vi "DBO.vi"(1 "H":dbl[][](array[numeric]), 2 "x":dbl) -> (0 "y":dbl)   [LabVIEW 2011]
uses:
  <vilib>/imath/engines/lvmath2/RunTimeEngine/ErrorHandling/NIMS_Finalize Error.vi
  <vilib>/imath/engines/lvmath2/RunTimeEngine/BuiltInFunctions/size/NIMS_I32=size(GM,I32).vi
  <instcachedir>/0/NIMS_I32=size(GM,I32)_C888250C35F946008B07D98778967D76.lvgen/NIMS_I32=size(GM,I32)_C888250C35F946008B07D98778967D76_004.vi
  <vilib>/imathl/engines/lvmath/Functions/Error Handling/Create Error.vi
  <vilib>/imath/engines/lvmath2/RunTimeEngine/CommandStatement/NIMS_CommandStatement_MaskErr.vi
  <vilib>/imath/engines/lvmath2/RunTimeEngine/VariableToken/NIMS_VariableToken_CondDefined.vi
  <instcachedir>/0/NIMS_VariableToken_CondDefined_D30D2F4D3CE04567BC79CC35D27951F7.lvgen/NIMS_VariableToken_CondDefined_D30D2F4D3CE04567BC79CC35D27951F7_003.vi
  <vilib>/imath/engines/lvmath/Functions/Error Handling/MergeErrorsWrapper.vi
  <vilib>/imath/engines/lvmath2/RunTimeEngine/NodeEndStatement/NIMS_NodeEndStatement_Output.vi
  <instcachedir>/0/NIMS_NodeEndStatement_Output_53EC0D466D134D7ABD903AC30B43404B.lvgen/NIMS_NodeEndStatement_Output_53EC0D466D134D7ABD903AC30B43404B_001.vi
  <vilib>/imath/engines/lvmath2/RunTimeEngine/VariableToken/Read/NIMS_Get Elements - SorM(_,_) - Check - Check.vi
  <instcachedir>/0/NIMS_Get Elements - SorM(_,_) - Check - Check_DA1E252EAB634D989357E7C72E8137F5.lvgen/NIMS_Get Elements - SorM(_,_) - Check - Check_DA1E252EAB634D989357E7C72E8137F5_001.vi
  C:/Documents and Settings/yna/My Documents/LabVIEW Data/MathScriptVIs/MCStatic_285220864_6d3d3726c5e701717503ad0a97b9c04b.vi
  <instcachedir>/0/MCStatic_285220864_6d3d3726c5e701717503ad0a97b9c04b_95A5838EAFCD4223B404CBD5C4A8267C.lvgen/MCStatic_285220864_6d3d3726c5e701717503ad0a97b9c04b_95A5838EAFCD4223B404CBD5C4A8267C_000.vi
  C:/Documents and Settings/yna/My Documents/LabVIEW Data/MathScriptVIs/MCStatic_285220864_904684f4bc757d8a144c5b0c95be3f99.vi
  <instcachedir>/0/MCStatic_285220864_904684f4bc757d8a144c5b0c95be3f99_DB46245F63EA4693B729F1F383828BBE.lvgen/MCStatic_285220864_904684f4bc757d8a144c5b0c95be3f99_DB46245F63EA4693B729F1F383828BBE_000.vi
  <vilib>/imath/engines/lvmath2/RunTimeEngine/BuiltInFunctions/min/2 inputs/NIMS_min(RG,RG)-no size check.vi
  <instcachedir>/0/NIMS_min(RG,RG)-no size check_7F67BAB91AFC452D9517D2EA1C8F5F88.lvgen/NIMS_min(RG,RG)-no size check_7F67BAB91AFC452D9517D2EA1C8F5F88_001.vi
  <vilib>/imath/engines/lvmath2/RunTimeEngine/CommandStatement/MC_CommandStatement_break.vi
  <vilib>/imath/engines/lvmath2/RunTimeEngine/ErrorHandling/NIMS_Create Error From Enums.vi
  <vilib>/imath/engines/lvmath2/RunTimeEngine/BuiltInFunctions/bitnot/NIMS_bitnot(SorS,SorS).vi
  <vilib>/imath/engines/lvmath2/RunTimeEngine/BuiltInFunctions/bitand/NIMS_bitand(SorS,SorS).vi
  <vilib>/imath/engines/lvmath2/RunTimeEngine/BuiltInFunctions/bitor/NIMS_bitor(SorS,SorS).vi
  f0.m
  f1.m
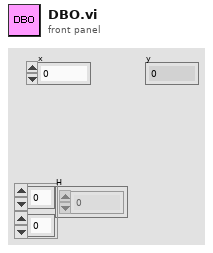
[diagram p1: front panel]
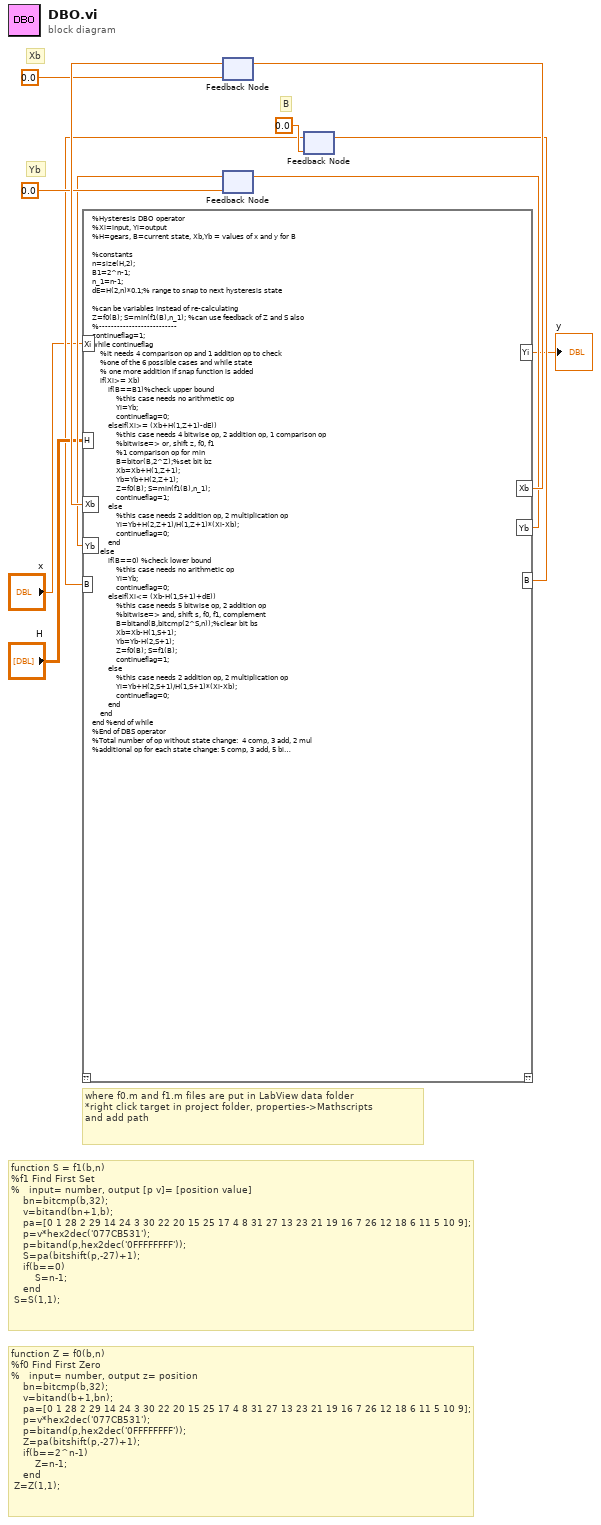
[diagram p0: block diagram]
diagram:
  # "function Z = f0(b,n)\n%f0 Find First Zero\n%   input= number, output z= position\n    bn=bitcmp(b,32);\n    v=bitand(b+1,bn);\n    pa=[0 1 28 2 29 14 24 3 30 22 20 15 25 17 4 8 31 27 13 23 21 19 16 7 26 12 18 6 11 5 10 9];\n    p=v*hex2dec('077CB531');\n    p=bitand(p,hex2dec('0FFFFFFFF'));\n    Z=pa(bitshift(p,-27)+1);\n    if(b==2^n-1) \n        Z=n-1;\n    end\n\tZ=Z(1,1);"
  # "function S = f1(b,n)\n%f1 Find First Set\n%   input= number, output [p v]= [position value]\n    bn=bitcmp(b,32);\n    v=bitand(bn+1,b);\n    pa=[0 1 28 2 29 14 24 3 30 22 20 15 25 17 4 8 31 27 13 23 21 19 16 7 26 12 18 6 11 5 10 9];\n    p=v*hex2dec('077CB531');\n    p=bitand(p,hex2dec('0FFFFFFFF'));\n    S=pa(bitshift(p,-27)+1);\n    if(b==0) \n        S=n-1;\n    end\n\tS=S(1,1);"
  # "where f0.m and f1.m files are put in LabView data folder\n*right click target in project folder, properties->Mathscripts\nand add path"
  # "B"
  # "Yb"
  # "Xb"
  n1 = feedback #1(0.0 ("Xk")) -> (w11:dbl)
  n2 = feedback #2(0.0 ("Xk")) -> (w7:dbl)
  n3 = feedback #3(0.0 ("Xk")) -> (w3:dbl)
  n4 = mathscript code="%Hysteresis DBO operator\n%Xi=input, Yi=output\n%H=gears, B=current state, Xb,Yb = values of x and y for B \n\n%constants\nn=size(H,2); \nB1=2^n-1; \nn_1=n-1;\ndE=H(2,n)*0.1;% range to snap to next hysteresis state\n\n%can be variables instead of re-calculating\nZ=f0(B); S=min(f1(B),n_1); %can use feedback of Z and S also\n%--------------------------\ncontinueflag=1;\nwhile continueflag\n    %it needs 4 comparison op and 1 addition op to check\n    %one of the 6 possible cases and while state\n    % one more addition if snap function is added\n    if(Xi>= Xb)  \n        if(B==B1)%check upper bound\n            %this case needs no arithmetic op\n            Yi=Yb;\n            continueflag=0;\n        elseif(Xi>= (Xb+H(1,Z+1)-dE))   \n            %this case needs 4 bitwise op, 2 addition op, 1 comparison op\n            %bitwise=> or, shift z, f0, f1\n            %1 comparison op for min\n            B=bitor(B,2^Z);%set bit bz\n            Xb=Xb+H(1,Z+1);\n            Yb=Yb+H(2,Z+1);  \n            Z=f0(B); S=min(f1(B),n_1); \n            continueflag=1;\n        else\n            %this case needs 2 addition op, 2 multiplication op\n            Yi=Yb+H(2,Z+1)/H(1,Z+1)*(Xi-Xb);\n            continueflag=0;\n        end\n    else\n        if(B==0) %check lower bound \n            %this case needs no arithmetic op\n            Yi=Yb;\n            continueflag=0;\n        elseif(Xi<= (Xb-H(1,S+1)+dE))\n            %this case needs 5 bitwise op, 2 addition op\n            %bitwise=> and, shift s, f0, f1, complement\n            B=bitand(B,bitcmp(2^S,n));%clear bit bs\n            Xb=Xb-H(1,S+1);\n            Yb=Yb-H(2,S+1); \n            Z=f0(B); S=f1(B); \n            continueflag=1;           \n        else\n            %this case needs 2 addition op, 2 multiplication op\n            Yi=Yb+H(2,S+1)/H(1,S+1)*(Xi-Xb);\n            continueflag=0;\n        end\n    end\nend %end of while\n%End of DBS operator\n%Total number of op without state change:  4 comp, 3 add, 2 mul\n%additional op for each state change: 5 comp, 3 add, 5 bitwise\n%--------------------------"("Xi"="x", "Xb"=w11, "Yb"=w7, "B"=w3, "H"="H") -> ("Yi"=→"y":dbl, "Xb"=w12:dbl, "Yb"=w8:dbl, "B"=w5:dbl)  [unwired: 1 in, 1 out]
  n5 = feedback-in #1(w12) -> ()
  n6 = feedback-in #2(w8) -> ()
  n7 = feedback-in #3(w5) -> ()
